vi "Get.vi"(11 "Управление ПЛК":T3) -> (0 "error out":errorcluster, 1 "Pair out":T1={"Давление заданное"=0.3, "Давление в системе"=99.99, "Расход заданый"=0.0, "Расход текущий"=0.0, "Объём заданный"=0.0, "Объём текущий"=0.0, "Старт давление"=FALSE, "Старт расход"=FALSE, "Сброс объёма"=FALSE, "plc_control"=FALSE, "lag_control"=FALSE, "mstop_control"=FALSE, "Давление"={"АЦП CH 0"=0.0, "АЦП CH 1"=0.0, "АЦП CH 2"=0.0, "АЦП CH 3"=0.0, "АЦП CH 4"=0.0, "АЦП CH 5"=0.0, "АЦП CH 6"=0.0, "АЦП CH 7"=0.0}, "Modbus"={"Массив чтения"=[], "Массив записи"=[]}} {"Давление"."АЦП CH 7" format="%.3f"; "Давление"."АЦП CH 6" format="%.3f"; "Давление"."АЦП CH 5" format="%.3f"; "Давление"."АЦП CH 4" format="%.3f"; "Давление"."АЦП CH 3" format="%.3f"; "Давление"."АЦП CH 2" format="%.3f"; "Давление"."АЦП CH 1" format="%.3f"; "Давление"."АЦП CH 0" format="%.3f"; "Объём текущий" min=0.0 max=9999.0 step=0.0001 format="%#_5f"; "Объём заданный" min=0.0 max=9999.0 step=0.0001 format="%#_5f"; "Расход текущий" format="%#_5f"; "Расход заданый" min=0.0 max=40.0 step=0.0001 format="%#_5f"; "Давление в системе" format="%.3f"; "Давление заданное" min=0.3 max=100.0 step=0.01 format="%#_5f"}, 2 "Port 2 out":T2={"Давление заданное"=0.3, "Давление MAX заданное"=100.0, "Давление в насосе"=0.0, "Давление в системе"=99.99, "Расход заданый"=0.0, "Расход текущий"=0.0, "Объём заданный"=0.0, "Объём текущий"=0.0, "Позиция насоса %"=0.0, "Ток двигателя"=0.0, "controlMsg"="", "Клапан k_sys"=FALSE, "Клапан k_res"=FALSE, "Клапан k_air"=FALSE, "Вверх"=FALSE, "Домой"=FALSE, "Вниз"=FALSE, "Старт расход"=FALSE, "Старт давление"=FALSE, "Сброс объёма"=FALSE, "Сброс давления Рсис"=FALSE, "Сброс давления Рнас"=FALSE, "Bits"={"plc_control"=FALSE, "lag_control"=FALSE, "mstop_control"=FALSE, "st_home"=FALSE, "error"=FALSE, "mstart"=FALSE, "pair"=FALSE, "startQ"=FALSE, "startP"=FALSE, "volume_Stop"=FALSE}} {"Ток двигателя" format="%#_5f"; "Расход текущий" format="%#_5f"; "Давление в системе" format="%.3f"; "Объём текущий" min=0.0 max=9999.0 step=0.0001 format="%#_5f"; "Объём заданный" min=0.0 max=9999.0 step=0.0001 format="%#_5f"; "Давление MAX заданное" min=0.0 max=100.0 step=0.01 format="%#_5f"; "Давление заданное" min=0.3 max=100.0 step=0.01 format="%#_5f"; "Расход заданый" min=0.0 max=40.0 step=0.0001 format="%#_5f"; "Давление в насосе" format="%.3f"; "Позиция насоса %" scale=0.0..100.0 scale format="%.2f"}, 3 "Port 1 out":T2={"Давление заданное"=0.3, "Давление MAX заданное"=100.0, "Давление в насосе"=0.0, "Давление в системе"=99.99, "Расход заданый"=0.0, "Расход текущий"=0.0, "Объём заданный"=0.0, "Объём текущий"=0.0, "Позиция насоса %"=0.0, "Ток двигателя"=0.0, "controlMsg"="", "Клапан k_sys"=FALSE, "Клапан k_res"=FALSE, "Клапан k_air"=FALSE, "Вверх"=FALSE, "Домой"=FALSE, "Вниз"=FALSE, "Старт расход"=FALSE, "Старт давление"=FALSE, "Сброс объёма"=FALSE, "Сброс давления Рсис"=FALSE, "Сброс давления Рнас"=FALSE, "Bits"={"plc_control"=FALSE, "lag_control"=FALSE, "mstop_control"=FALSE, "st_home"=FALSE, "error"=FALSE, "mstart"=FALSE, "pair"=FALSE, "startQ"=FALSE, "startP"=FALSE, "volume_Stop"=FALSE}} {"Ток двигателя" format="%#_5f"; "Расход текущий" format="%#_5f"; "Давление в системе" format="%.3f"; "Объём текущий" min=0.0 max=9999.0 step=0.0001 format="%#_5f"; "Объём заданный" min=0.0 max=9999.0 step=0.0001 format="%#_5f"; "Давление MAX заданное" min=0.0 max=100.0 step=0.01 format="%#_5f"; "Давление заданное" min=0.3 max=100.0 step=0.01 format="%#_5f"; "Расход заданый" min=0.0 max=40.0 step=0.0001 format="%#_5f"; "Давление в насосе" format="%.3f"; "Позиция насоса %" scale=0.0..100.0 scale format="%.2f"})   [LabVIEW 2023, in "pump_Lib.lvlib"]
uses:
  pump_Lib.lvlib
  TypeDef/control_Type.ctl
  TypeDef/pump_Type.ctl
  TypeDef/pair_Type.ctl
  TypeDef/parametrs_Type.ctl
panel:
  # "%"
  # "%"
  # "%"
  # "%"
  # "%"
  # "%"
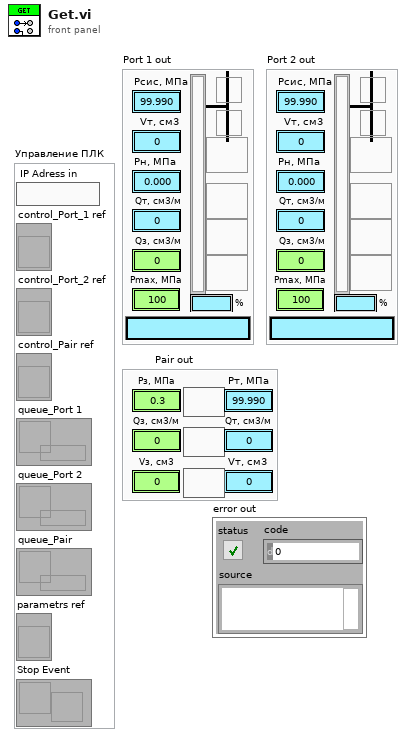
[diagram p1: front panel]
types:
  T1 = typedef "pump_Lib.lvlib/pair_Type.ctl" = cluster{"Давление заданное":dbl, "Давление в системе":dbl, "Расход заданый":dbl, "Расход текущий":dbl, "Объём заданный":dbl, "Объём текущий":dbl, "Старт давление":bool, "Старт расход":bool, "Сброс объёма":bool, "plc_control":bool, "lag_control":bool, "mstop_control":bool, "Давление":cluster{"АЦП CH 0":dbl, "АЦП CH 1":dbl, "АЦП CH 2":dbl, "АЦП CH 3":dbl, "АЦП CH 4":dbl, "АЦП CH 5":dbl, "АЦП CH 6":dbl, "АЦП CH 7":dbl}, "Modbus":cluster{"Массив чтения":u16[], "Массив записи":u16[]}}
  T2 = typedef "pump_Lib.lvlib/pump_Type.ctl" = cluster{"Давление заданное":dbl, "Давление MAX заданное":dbl, "Давление в насосе":dbl, "Давление в системе":dbl, "Расход заданый":dbl, "Расход текущий":dbl, "Объём заданный":dbl, "Объём текущий":dbl, "Позиция насоса %":dbl, "Ток двигателя":dbl, "controlMsg":string, "Клапан k_sys":bool, "Клапан k_res":bool, "Клапан k_air":bool, "Вверх":bool, "Домой":bool, "Вниз":bool, "Старт расход":bool, "Старт давление":bool, "Сброс объёма":bool, "Сброс давления Рсис":bool, "Сброс давления Рнас":bool, "Bits":cluster{"plc_control":bool, "lag_control":bool, "mstop_control":bool, "st_home":bool, "error":bool, "mstart":bool, "pair":bool, "startQ":bool, "startP":bool, "volume_Stop":bool}}
  T3 = typedef "pump_Lib.lvlib/control_Type.ctl" = cluster{"IP Adress in":string, "control_Port_1 ref":refnum<vi>, "control_Port_2 ref":refnum<vi>, "control_Pair ref":refnum<vi>, "queue_Port 1":refnum<queue>, "queue_Port 2":refnum<queue>, "queue_Pair":refnum<queue>, "parametrs ref":refnum<vi>, "Stop Event":refnum<user-event>}
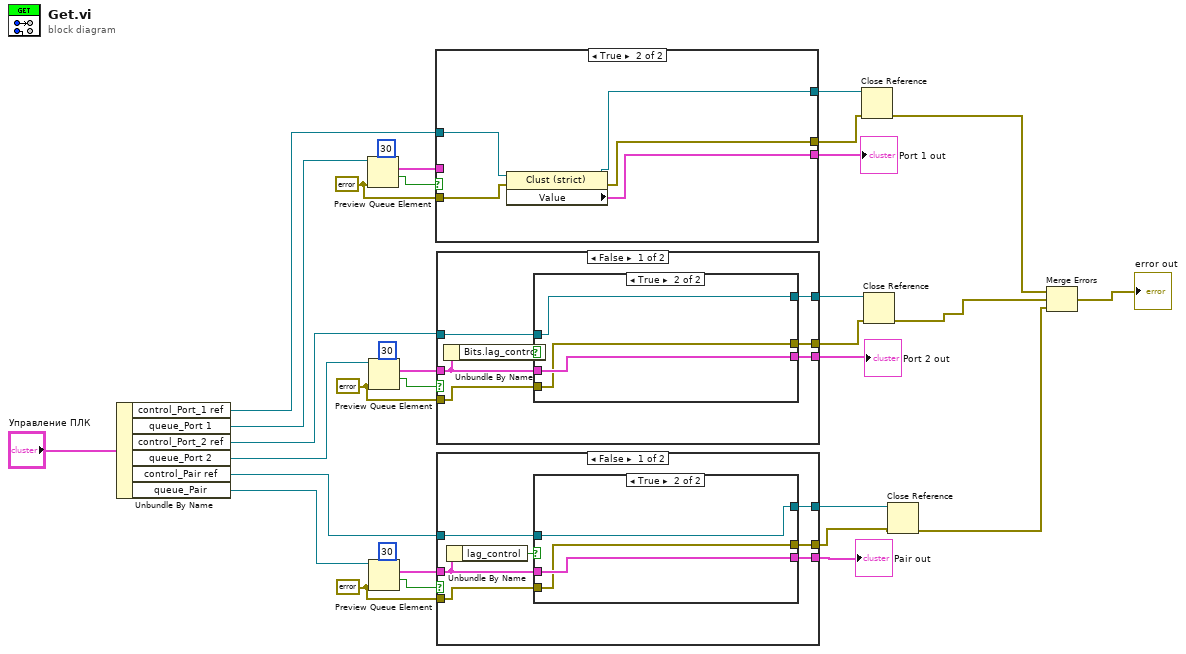
[diagram p0: block diagram]
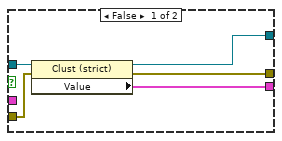
[diagram p2: hidden frame]
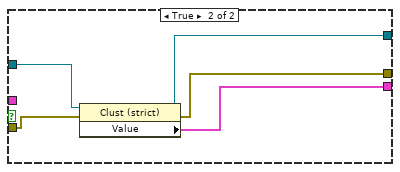
[diagram p3: hidden frame]
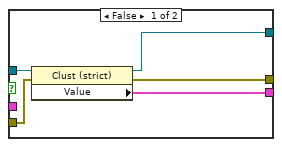
[diagram p4: hidden frame]
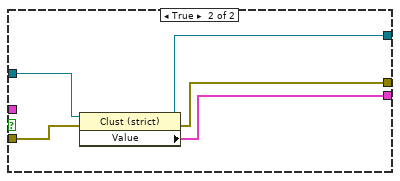
[diagram p5: hidden frame]
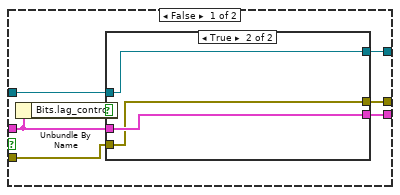
[diagram p6: hidden frame]
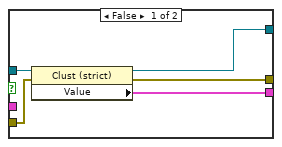
[diagram p7: hidden frame]
diagram:
  w12 = errorcluster {"status"=FALSE, "code"=0, "source"=""} ("error in (no error)")
  w14 = errorcluster {"status"=FALSE, "code"=0, "source"=""} ("error in (no error)")
  w15 = errorcluster {"status"=FALSE, "code"=0, "source"=""} ("error in (no error)")
  n1 = Unbundle By Name("Управление ПЛК") -> ("control_Port_1 ref"=w29:refnum<vi>, "queue_Port 1"=w28:refnum<queue>, "control_Port_2 ref"=w25:refnum<vi>, "queue_Port 2"=w24:refnum<queue>, "control_Pair ref"=w20:refnum<vi>, "queue_Pair"=w19:refnum<queue>)
  n2 = Preview Queue Element(queue=w28, timeout in ms (-1)=30, error in (no error)=w15) -> (element=w31:T2, timed out?=w16:bool)  [unwired: 2 out]
  n3 = Preview Queue Element(queue=w24, timeout in ms (-1)=30, error in (no error)=w14) -> (element=w26:T2, timed out?=w13:bool)  [unwired: 2 out]
  n4 = Preview Queue Element(queue=w19, timeout in ms (-1)=30, error in (no error)=w12) -> (element=w22:T1, timed out?=w11:bool)  [unwired: 2 out]
  n5 = case shown="True" w16 {
    tunnel: w31 -> [w36 _]
    tunnel: [w38 w50] -> w17
    tunnel: [w39 w52] -> w6
    tunnel: w29 -> [w35 w51]
    tunnel: w15 -> [w34 w49]
    tunnel: [w33 w48] -> w5
    frame False {
      n6 = Unbundle By Name(w36) -> ("Bits.lag_control"=w37:bool)
      n7 = case shown="True" w37 {
        tunnel: w36 -> [_ w47]
        tunnel: [w44 w47] -> w38
        tunnel: [w41 w46] -> w39
        tunnel: w34 -> [w42 w46]
        tunnel: w35 -> [w43 w45]
        tunnel: [w40 w45] -> w33
        frame False {
          n8 = property class="Clust (strict)"(reference=w43, error in=w42) -> (reference out=w40:refnum<vi>, error out=w41:errorcluster, "Value"=w44:T2)
        }
        frame True {
        }
      }
    }
    frame True {
      n9 = property class="Clust (strict)"(reference=w51, error in=w49) -> (reference out=w48:refnum<vi>, error out=w52:errorcluster, "Value"=w50:T2)
    }
  }
  "Port 1 out" <- w17
  n10 = case shown="False" w13 {
    tunnel: w26 -> [w56 _]
    tunnel: [w58 w70] -> w18
    tunnel: [w59 w72] -> w8
    tunnel: w25 -> [w55 w71]
    tunnel: w14 -> [w54 w69]
    tunnel: [w53 w68] -> w7
    frame False {
      n11 = Unbundle By Name(w56) -> ("Bits.lag_control"=w57:bool)
      n12 = case shown="True" w57 {
        tunnel: w56 -> [_ w67]
        tunnel: [w64 w67] -> w58
        tunnel: [w62 w66] -> w59
        tunnel: w54 -> [w61 w66]
        tunnel: w55 -> [w63 w65]
        tunnel: [w60 w65] -> w53
        frame False {
          n13 = property class="Clust (strict)"(reference=w63, error in=w61) -> (reference out=w60:refnum<vi>, error out=w62:errorcluster, "Value"=w64:T2)
        }
        frame True {
        }
      }
    }
    frame True {
      n14 = property class="Clust (strict)"(reference=w71, error in=w69) -> (reference out=w68:refnum<vi>, error out=w72:errorcluster, "Value"=w70:T2)
    }
  }
  "Port 2 out" <- w18
  n15 = case shown="False" w11 {
    tunnel: w22 -> [w76 _]
    tunnel: [w78 w90] -> w21
    tunnel: [w79 w92] -> w10
    tunnel: w20 -> [w75 w91]
    tunnel: w12 -> [w74 w89]
    tunnel: [w73 w88] -> w9
    frame False {
      n16 = Unbundle By Name(w76) -> ("lag_control"=w77:bool)
      n17 = case shown="True" w77 {
        tunnel: w76 -> [_ w87]
        tunnel: [w84 w87] -> w78
        tunnel: [w81 w86] -> w79
        tunnel: w74 -> [w83 w86]
        tunnel: w75 -> [w82 w85]
        tunnel: [w80 w85] -> w73
        frame False {
          n18 = property class="Clust (strict)"(reference=w82, error in=w83) -> (reference out=w80:refnum<vi>, error out=w81:errorcluster, "Value"=w84:T1)
        }
        frame True {
        }
      }
    }
    frame True {
      n19 = property class="Clust (strict)"(reference=w91, error in=w89) -> (reference out=w88:refnum<vi>, error out=w92:errorcluster, "Value"=w90:T1)
    }
  }
  "Pair out" <- w21
  n20 = Close Reference(reference=w5, error in (no error)=w6) -> (error out=w4:errorcluster)
  n21 = Close Reference(reference=w7, error in (no error)=w8) -> (error out=w2:errorcluster)
  n22 = Close Reference(reference=w9, error in (no error)=w10) -> (error out=w1:errorcluster)
  n23 = Merge Errors(w4, w2, w1) -> (→"error out":errorcluster)
